vi "Get Material Name from Serial Number.vi"(6 "Engineering Mode":bool, 9 "Material Type Reference":string, 10 "Serial Number":string, 11 "Application in":refnum<class "Application.lvclass">) -> (0 "error out":errorcluster, 1 "Material Type out":string, 2 "Gold Board":bool, 3 "Next State":string)   [LabVIEW 2017, in "Application.lvlib" / "Application.lvclass"]
doc: "Attempts to retrieve the material type from an MES DB based on the serial number. If unavailable, returns an error unless user is logged in as admin, which will prompt for serial. If MES is disabled, always prompts."
uses:
  Application.lvclass
  Test Recipe/Class/Test Recipe.lvclass
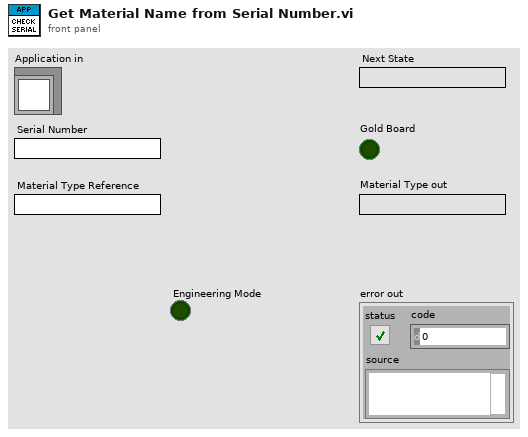
[diagram p1: front panel]
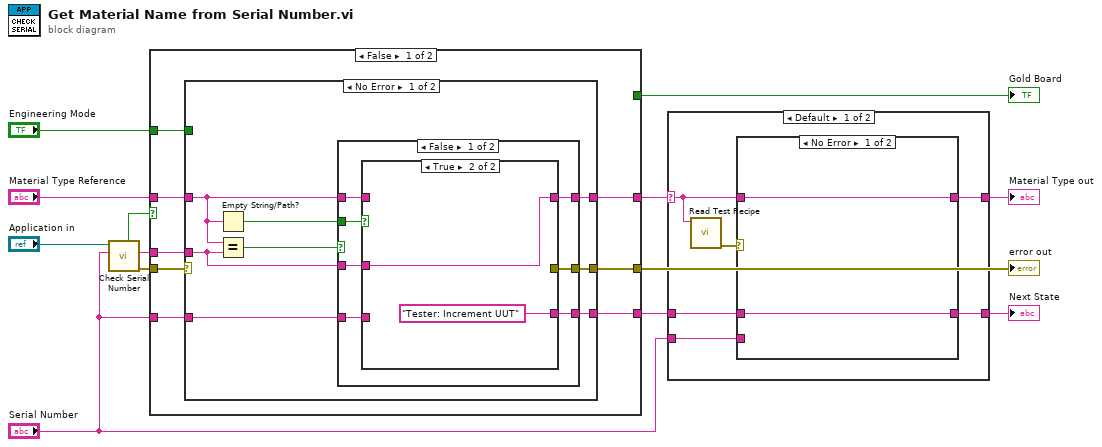
[diagram p0: block diagram]
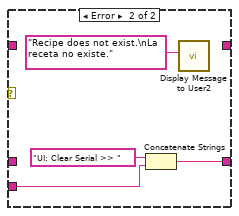
[diagram p2: hidden frame]
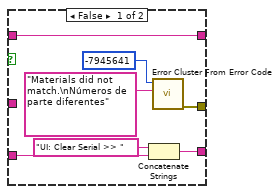
[diagram p4: hidden frame]
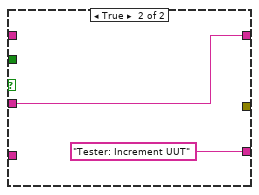
[diagram p5: hidden frame]
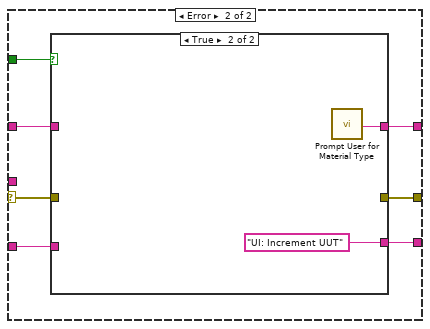
[diagram p6: hidden frame]
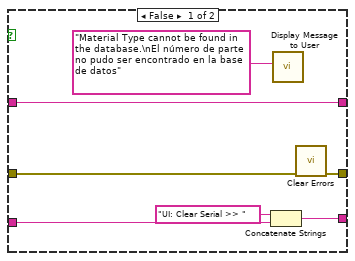
[diagram p7: hidden frame]
diagram:
  n1 = call "Check Serial Number.vi"("Serial ID"="Serial Number", "Application in"="Application in") -> ("error out"=w10:errorcluster, "Material Type"=w11:string, "Gold Board"=w12:bool)  [unwired: 6 in, 1 out]
  n2 = case shown="False" w12 {
    selector: w12 -> [_ w64]
    tunnel: "Engineering Mode" -> [w17 _]
    tunnel: [w21 _] -> w13
    tunnel: w11 -> [w20 w65]
    tunnel: [w19 w65] -> w6
    tunnel: w10 -> [w18 _]
    tunnel: "Material Type Reference" -> [w16 _]
    tunnel: "Serial Number" -> [w15 _]
    tunnel: [w14 _] -> w4
    tunnel: [_ w64] -> w1
    frame False {
      n3 = case shown="No Error" w18 {
        selector: w18 -> [_ w53]
        tunnel: [w27 w52] -> w21
        tunnel: w20 -> [w26 _]
        tunnel: [w25 w51] -> w19
        tunnel: w17 -> [_ w54]
        tunnel: w16 -> [w24 w50]
        tunnel: w15 -> [w23 w49]
        tunnel: [w22 w48] -> w14
        frame No Error {
          n4 = Empty String/Path?(string/path=w24) -> (empty?=w28:bool)
          n5 = Equal?(x=w24, y=w26) -> (x = y?=w29:bool)
          n6 = case shown="False" w29 {
            tunnel: w26 -> [w34 w47]
            tunnel: [w33 w47] -> w25
            tunnel: w24 -> [w36 _]
            tunnel: w28 -> [w35 _]
            tunnel: [w32 _] -> w27
            tunnel: w23 -> [w31 _]
            tunnel: [w30 "Tester: Increment UUT" ("State(s) at Back (\"\")")] -> w22
            frame False {
              n7 = case shown="True" w35 {
                tunnel: w36 -> [w43 _]
                tunnel: w34 -> [_ w45]
                tunnel: [w43 w45] -> w33
                tunnel: [w42 _] -> w32
                tunnel: w31 -> [w38 _]
                tunnel: [w37 "Tester: Increment UUT" ("State(s) at Back (\"\")")] -> w30
                frame False {
                  n8 = Concatenate Strings("UI: Clear Serial >> " ("State(s) at Back (\"\")"), w38) -> (w37:string)
                  n9 = call <vilib>:"Error Cluster From Error Code.vi"("error message (\"\")"="Materials did not match.\nNúmeros de parte diferentes" ("error message (\"\")"), "error code (0)"=-7945641) -> ("error out"=w42:errorcluster)  [unwired: 7 in]
                }
                frame True {
                }
              }
            }
            frame True {
            }
          }
        }
        frame Error {
          n10 = case shown="True" w54 {
            tunnel: w53 -> [w61 _]
            tunnel: [w58 _] -> w52
            tunnel: [w60 w63] -> w51
            tunnel: w50 -> [w60 _]
            tunnel: w49 -> [w56 _]
            tunnel: [w55 "UI: Increment UUT" ("State(s) at Back (\"\")")] -> w48
            frame False {
              n11 = Concatenate Strings("UI: Clear Serial >> " ("State(s) at Back (\"\")"), w56) -> (w55:string)
              n12 = call "Display Message to User"("Message"="Material Type cannot be found in the database.\nEl número de parte no pudo ser encontrado en la base de datos") -> ()  [unwired: 9 in, 2 out]
              n13 = call <vilib>:"Clear Errors.vi"("error in (no error)"=w61) -> ("error out"=w58:errorcluster)  [unwired: 5 in, 1 out]
            }
            frame True {
              n14 = call "Prompt User for Material Type"() -> ("Material Type"=w63:string)  [unwired: 17 in, 2 out]
            }
          }
        }
      }
    }
    frame True {
    }
  }
  "error out" <- w13
  "Gold Board" <- w1
  n15 = case shown="Default" w6 {
    selector: w6 -> [w69 w79]
    tunnel: [w70 w79] -> w5
    tunnel: w4 -> [w67 w78]
    tunnel: [w68 w78] -> w3
    tunnel: "Serial Number" -> [w66 _]
    frame Default {
      n16 = call "Read Test Recipe.vi"("Material Type"=w69) -> ("error out"=w71:errorcluster)  [unwired: 9 in, 1 out]
      n17 = case shown="No Error" w71 {
        tunnel: [w73 _] -> w70
        tunnel: w69 -> [w73 _]
        tunnel: [w72 w75] -> w68
        tunnel: w67 -> [w72 _]
        tunnel: w66 -> [_ w76]
        frame No Error {
        }
        frame Error {
          n18 = Concatenate Strings("UI: Clear Serial >> " ("State(s) at Back (\"\")"), w76) -> (w75:string)
          n19 = call "Display Message to User2"("Message"="Recipe does not exist.\nLa receta no existe.") -> ()  [unwired: 9 in, 2 out]
        }
      }
    }
    frame "" {
    }
  }
  "Next State" <- w3
  "Material Type out" <- w5
